vi "Device Select.vi"(8 "error in":errorcluster, 10 "SQL query":string="SELECT distinct DeviceName\n FROM ltt.daq_configuration \nWhere ChannelType='Analog_Input' and Enabled=1;", 11 "NI Analog Input in":refnum<class "NI Analog Input.lvclass">) -> (0 "error out":errorcluster, 3 "NI Analog Input out":refnum<class "NI Analog Input.lvclass">)   [LabVIEW 2023, in "HardwareAbstractionLayer_LVOOP.lvlib" / "NI Analog Input.lvclass"]
doc: "This VI is Device Select"
uses:
  NI Analog Input.lvclass
  NI Analog Input.lvclass/NI Analog Input.ctl
  Database/Database.lvclass
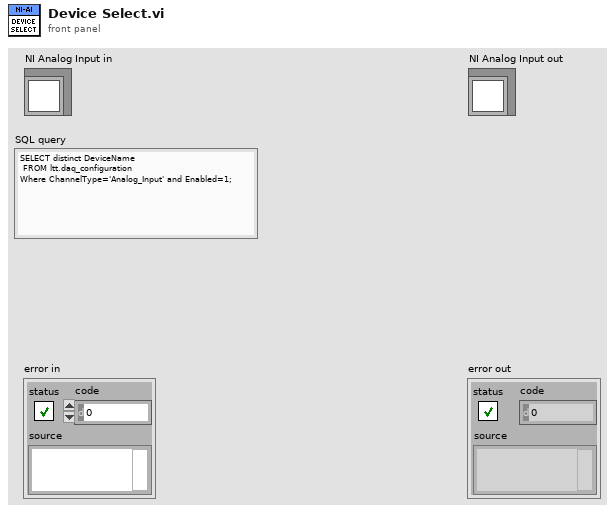
[diagram p1: front panel]
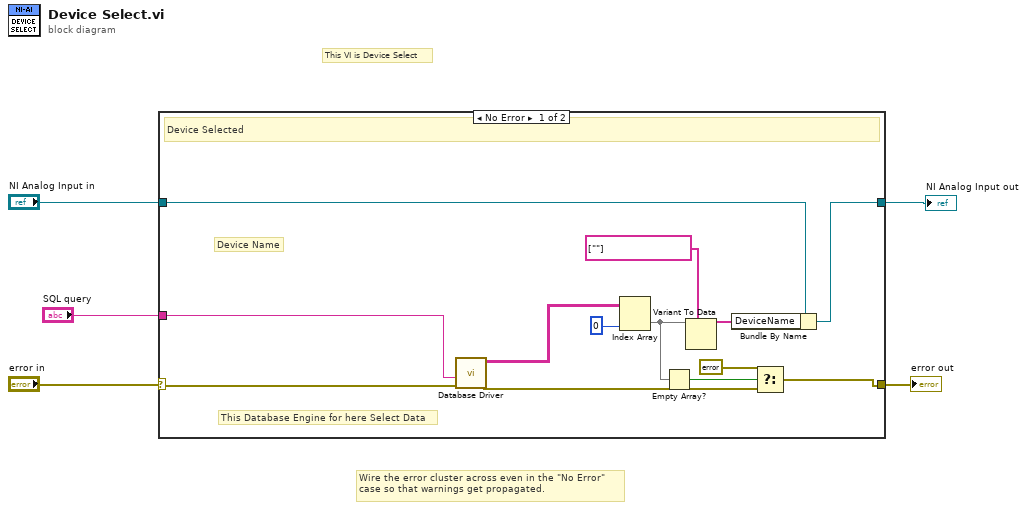
[diagram p0: block diagram]
diagram:
  # "This VI is Device Select"
  # "Wire the error cluster across even in the \"No Error\"\ncase so that warnings get propagated."
  n1 = case shown="No Error" "error in" {
    selector: "error in" -> [w13 w20]
    tunnel: [w7 w20] -> w4
    tunnel: [w17 w19] -> w2
    tunnel: "NI Analog Input in" -> [w18 w19]
    tunnel: "SQL query" -> [w11 _]
    frame No Error {
      # "This Database Engine for here Select Data"
      # "Device Name"
      # "Device Selected"
      n2 = call "Database Driver.vi"("error in"=w13, "SQL query"=w11) -> ("error out"=w8:errorcluster, "data"=w12:string[][])  [unwired: 6 in, 2 out]
      n3 = Index Array(array=w12, index (col)=0 ("disabled index (col)")) -> (element=w10:string[])  [unwired: 1 in]
      n4 = Empty Array?(array=w10) -> (empty?=w9:bool)
      n5 = Variant To Data(type=tag[] [""] ("DeviceName"), Variant=w10) -> (data=w15:tag[])  [unwired: 1 in, 1 out]
      n6 = Bundle By Name(cluster=w18, "DeviceName"=w15) -> (w17:refnum<class "NI Analog Input.lvclass">)
      n7 = Select(t=errorcluster {"status"=TRUE, "code"=0, "source"="Database does not contains device which is query."}, s=w9, f=w8) -> (s? t:f=w7:errorcluster)
    }
    frame Error {
    }
  }
  "error out" <- w4
  "NI Analog Input out" <- w2
